vi "SteppertestLOWLEVEL.vi"() -> ()   [LabVIEW 2018]
uses:
  <vilib>/myRIO/Common/Instrument Driver Framework/myRIO v1.0/DIO/typedefs/DIO Channels Enum.ctl
  <vilib>/myRIO/Common/Instrument Driver Framework/myRIO v1.0/DIO/typedefs/DIO Channels List.ctl
  <vilib>/myRIO/Common/Instrument Driver Framework/Utilities/typedefs/Generic FPGA Reference.ctl
  <vilib>/myRIO/Common/Instrument Driver Framework/Utilities/typedefs/myRIO v1.0 Reference.ctl
  <vilib>/myRIO/Common/Instrument Driver Framework/Utilities/typedefs/Hardware Version Enum.ctl
  <vilib>/myRIO/Common/Instrument Driver Framework/Utilities/typedefs/myRIO Generic Hardware Reference.ctl
  <vilib>/myRIO/Instrument Drivers/Onboard IO/DIO/typedefs/DIO Reference.ctl
  <vilib>/myRIO/Instrument Drivers/Onboard IO/DIO/DIO.lvlib
  <vilib>/myRIO/Instrument Drivers/Onboard IO/DIO/vis/myRIO DIO Open.xnode
  <vilib>/myRIO/Common/Instrument Driver Framework/myRIO v1.0/DIO/vis/myRIO v1.1 Open DIO.vi
  <vilib>/userdefined/High Color/nirio_resource_hc.ctl
  <vilib>/myRIO/Instrument Drivers/Onboard IO/PWM/typedefs/PWM Configuration.ctl
  <vilib>/myRIO/Instrument Drivers/Onboard IO/PWM/PWM.lvlib
  <vilib>/myRIO/Common/Instrument Driver Framework/myRIO v1.0/PWM/typedefs/PWM Channels Enum.ctl
  <vilib>/myRIO/Instrument Drivers/Onboard IO/PWM/typedefs/PWM Reference.ctl
  <vilib>/myRIO/Instrument Drivers/Onboard IO/PWM/vis/myRIO PWM Open.xnode
  <vilib>/myRIO/Common/Instrument Driver Framework/myRIO v1.0/PWM/vis/myRIO v1.1 Open PWM.vi
  <vilib>/myRIO/Instrument Drivers/Utilities/Utilities.lvlib
panel:
  in  "DIR":bool
  in  "ENABLE":bool=TRUE
  in  "Frequency [Hz]":dbl=200.0
  in  "Duty Cycle":dbl
  in  "stop":bool
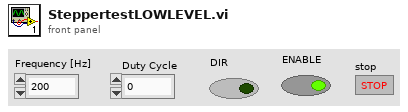
[diagram p1: front panel]
types:
  T1 = typedef "nirio_resource_hc.ctl" = tag
  T2 = typedef "Hardware Version Enum.ctl" = enum16{"Unknown", "myRIO-1900", "myRIO-1950", "roboRIO", "NI ELVIS RIO CM", "ELVIS III"}
  T3 = typedef "PWM.lvlib/PWM Reference.ctl" = cluster{"myRIO Reference":T4, "PWM Channels Enum":T7, "PWM Configuration":T8}
  T4 = typedef "myRIO Generic Hardware Reference.ctl" = cluster{"myRIO Model":T2, "myRIO Hardware Reference":T5}
  T5 = typedef "myRIO v1.0 Reference.ctl" = cluster{"Generic FPGA Reference":T6, "Allow multiple opens":bool}
  T6 = typedef "Generic FPGA Reference.ctl" = refnum<k20>
  T7 = typedef "PWM Channels Enum.ctl" = enum16{"Not Connected", "C/PWM0", "C/PWM1", "A/PWM0", "A/PWM1", "A/PWM2", "A/PWM3", "A/PWM4", "A/PWM5", "A/PWM6", "A/PWM7", "A/PWM8", "A/PWM9", "A/PWM10", "A/PWM11", "A/PWM12", "A/PWM13", "A/PWM14", "A/PWM15", "A/PWM16", "A/PWM17", "A/PWM18", "A/PWM19", "B/PWM0", "B/PWM1", "B/PWM2", "B/PWM3", "B/PWM4", "B/PWM5", "B/PWM6", "B/PWM7", "B/PWM8", "B/PWM9", "B/PWM10", "B/PWM11", "B/PWM12", "B/PWM13", "B/PWM14", "B/PWM15", "B/PWM16", "B/PWM17", "B/PWM18", "B/PWM19", "PWM/PWM0", "PWM/PWM1", "PWM/PWM2", "PWM/PWM3", "PWM/PWM4", "PWM/PWM5", "PWM/PWM6", "PWM/PWM7", "PWM/PWM8", "PWM/PWM9"}
  T8 = typedef "PWM.lvlib/PWM Configuration.ctl" = cluster{"Frequency":dbl, "Duty Cycle":dbl}
  T9 = typedef "DIO.lvlib/DIO Reference.ctl" = cluster{"myRIO Reference":T4, "DIO Channels List":T10}
  T10 = typedef "DIO Channels List.ctl" = T11[]
  T11 = typedef "DIO Channels Enum.ctl" = enum16{"Not Connected", "C/DIO0", "C/DIO1", "C/DIO2", "C/DIO3", "C/DIO4", "C/DIO5", "C/DIO6", "C/DIO7", "A/DIO0", "A/DIO1", "A/DIO2", "A/DIO3", "A/DIO4", "A/DIO5", "A/DIO6", "A/DIO7", "A/DIO8", "A/DIO9", "A/DIO10", "A/DIO11", "A/DIO12", "A/DIO13", "A/DIO14", "A/DIO15", "A/DIO16", "A/DIO17", "A/DIO18", "A/DIO19", "B/DIO0", "B/DIO1", "B/DIO2", "B/DIO3", "B/DIO4", "B/DIO5", "B/DIO6", "B/DIO7", "B/DIO8", "B/DIO9", "B/DIO10", "B/DIO11", "B/DIO12", "B/DIO13", "B/DIO14", "B/DIO15", "B/DIO16", "B/DIO17", "B/DIO18", "B/DIO19", "LED0", "LED1", "LED2", "LED3", "Button0", "DIO/DIO0", "DIO/DIO1", "DIO/DIO2", "DIO/DIO3", "DIO/DIO4", "DIO/DIO5", "DIO/DIO6", "DIO/DIO7", "DIO/DIO8", "DIO/DIO9", "SPI/CS0", "SPI/CS1", "SPI/CS2", "SPI/CS3", "LED RADIO (Green)", "LED RADIO (Red)", "LED COMM (Green)", "LED COMM (Red)", "LED MODE (Green)", "LED MODE (Red)"}
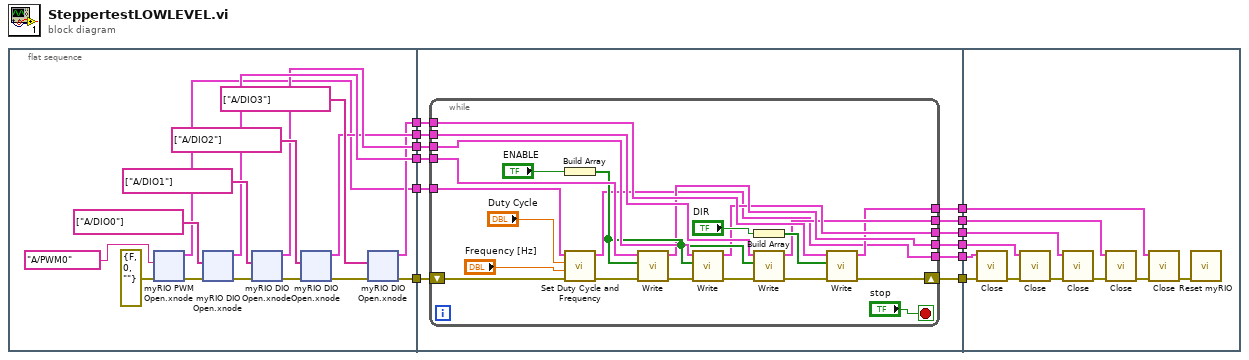
[diagram p0: block diagram]
diagram:
  n1 = flat-sequence {
    tunnel: [w18] -> w12
    tunnel: [w17] -> w11
    tunnel: [w16] -> w10
    tunnel: [w15] -> w9
    tunnel: [w14] -> w8
    tunnel: [w13] -> w1
    tunnel: w12 -> [w120]
    tunnel: w11 -> [w119]
    tunnel: w10 -> [w118]
    tunnel: w9 -> [w117]
    tunnel: w8 -> [w116]
    tunnel: [w115] -> w7
    tunnel: [w114] -> w6
    tunnel: [w113] -> w5
    tunnel: [w112] -> w4
    tunnel: [w111] -> w3
    tunnel: [w110] -> w2
    tunnel: w1 -> [w109]
    tunnel: w7 -> [w154]
    tunnel: w6 -> [w153]
    tunnel: w5 -> [w152]
    tunnel: w4 -> [w151]
    tunnel: w3 -> [w150]
    tunnel: w2 -> [w149]
    frame #0 {
      n2 = xnode "myRIO PWM Open.xnode"("error in (no error)"=errorcluster {"status"=FALSE, "code"=0, "source"=""} ("error constant"), "Channel Name"=tag "A/PWM0") -> ("error out"=w25:errorcluster, "PWM Ref Out"=w13:T3)  [unwired: 1 in]
      n3 = xnode "myRIO DIO Open.xnode"("error in (no error)"=w25, "Channel Names"=tag[] ["A/DIO0"]) -> ("error out"=w21:errorcluster, "DIO Ref Out"=w17:T9)  [unwired: 1 in]
      n4 = xnode "myRIO DIO Open.xnode"("error in (no error)"=w21, "Channel Names"=tag[] ["A/DIO1"]) -> ("error out"=w20:errorcluster, "DIO Ref Out"=w16:T9)  [unwired: 1 in]
      n5 = xnode "myRIO DIO Open.xnode"("error in (no error)"=w20, "Channel Names"=tag[] ["A/DIO2"]) -> ("error out"=w19:errorcluster, "DIO Ref Out"=w15:T9)  [unwired: 1 in]
      n6 = xnode "myRIO DIO Open.xnode"("error in (no error)"=w19, "Channel Names"=tag[] ["A/DIO3"]) -> ("error out"=w18:errorcluster, "DIO Ref Out"=w14:T9)  [unwired: 1 in]
    }
    frame #1 {
      n7 = while {
        tunnel: w119 -> [w140]
        tunnel: w118 -> [w139]
        tunnel: w117 -> [w138]
        tunnel: w116 -> [w133]
        tunnel: [w127] -> w115
        tunnel: [w126] -> w114
        tunnel: [w125] -> w113
        tunnel: [w124] -> w112
        tunnel: [w123] -> w111
        shift-right: [w122] -> w110
        shift-left: w120 -> [w132]
        tunnel: w109 -> [w121]
        stop <- "stop" stop-if-true
        n8 = Build Array("ENABLE") -> (w136:bool[])
        n9 = call <vilib>:"Set Duty Cycle and Frequency.vi"("error in (no error)"=w132, "Frequency [Hz]"="Frequency [Hz]", "Duty Cycle"="Duty Cycle", "PWM Ref In"=w121) -> ("error out"=w131:errorcluster, "PWM Ref Out"=w123:T3)  [unwired: 5 in]
        n10 = call <vilib>:"Write.vi"("error in (no error)"=w131, "Values"=w136, "DIO Ref In"=w140) -> ("error out"=w130:errorcluster, "DIO Ref Out"=w127:T9)  [unwired: 6 in]
        n11 = call <vilib>:"Write.vi"("error in (no error)"=w130, "Values"=w136, "DIO Ref In"=w139) -> ("error out"=w129:errorcluster, "DIO Ref Out"=w126:T9)  [unwired: 6 in]
        n12 = Build Array("DIR") -> (w134:bool[])
        n13 = call <vilib>:"Write.vi"("error in (no error)"=w129, "Values"=w136, "DIO Ref In"=w138) -> ("error out"=w128:errorcluster, "DIO Ref Out"=w125:T9)  [unwired: 6 in]
        n14 = call <vilib>:"Write.vi"("error in (no error)"=w128, "Values"=w134, "DIO Ref In"=w133) -> ("error out"=w122:errorcluster, "DIO Ref Out"=w124:T9)  [unwired: 6 in]
      }
    }
    frame #2 {
      n15 = call <vilib>:"Close.vi"("error in (no error)"=w149, "PWM Ref In"=w150) -> ("error out"=w148:errorcluster)  [unwired: 9 in]
      n16 = call <vilib>:"Close.vi"("error in (no error)"=w148, "DIO Ref In"=w154) -> ("error out"=w147:errorcluster)  [unwired: 9 in]
      n17 = call <vilib>:"Close.vi"("error in (no error)"=w147, "DIO Ref In"=w153) -> ("error out"=w146:errorcluster)  [unwired: 9 in]
      n18 = call <vilib>:"Close.vi"("error in (no error)"=w146, "DIO Ref In"=w152) -> ("error out"=w145:errorcluster)  [unwired: 9 in]
      n19 = call <vilib>:"Close.vi"("error in (no error)"=w145, "DIO Ref In"=w151) -> ("error out"=w144:errorcluster)  [unwired: 9 in]
      n20 = call <vilib>:"Reset myRIO.vi"("error in (no error)"=w144) -> ()  [unwired: 10 in, 1 out]
    }
  }
